vi "processTask.vi"(6 "taskChannelType":T1, 8 "error in (no error)":errorcluster, 11 "classPath":path) -> (0 "error out":errorcluster, 3 "classPath(dup)":path)   [LabVIEW 2023]
uses:
  stopMechanismType.ctl
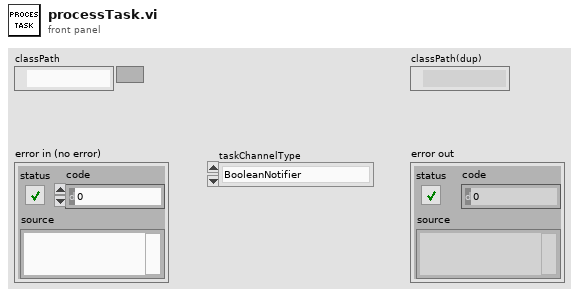
[diagram p1: front panel]
types:
  T1 = typedef "stopMechanismType.ctl" = enum16{"BooleanNotifier", "BooleanUE", "MsgUE", "MsgQueue"}
  T2 = cluster{"placeholderName":string, "filename without extension":string}
  T3 = cluster{"placeholderName":string, "filename without extension":string}[]
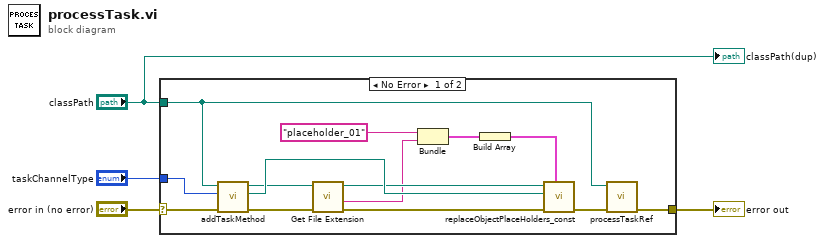
[diagram p0: block diagram]
diagram:
  n1 = case shown="No Error" "error in (no error)" {
    selector: "error in (no error)" -> [w18 w19]
    tunnel: "classPath" -> [w5 _]
    tunnel: [w6 w19] -> w3
    tunnel: "taskChannelType" -> [w15 _]
    frame No Error {
      n2 = call "addTaskMethod.vi"("error in"=w18, "stopMechanismType"=w15, "classPath"=w5) -> ("error out"=w12:errorcluster, "taskViPath"=w16:path, "classPath(dup)"=w10:path)  [unwired: 6 in]
      n3 = call <vilib>:"Get File Extension.vi"("error in (no error)"=w12, "file"=w10) -> ("error out"=w11:errorcluster, "filename without extension"=w8:string, "dup file"=w9:path)  [unwired: 5 in, 2 out]
      n4 = Bundle("placeholderName"="placeholder_01", "filename without extension"=w8) -> (w14:T2)  [unwired: 1 in]
      n5 = Build Array(w14) -> (w13:T3)
      n6 = call "replaceObjectPlaceHolders_const.vi"("placeholderList"=w13, "error in (no error)"=w11, "targetVI"=w16, "classPathToReplace"=w9) -> ("error out"=w7:errorcluster)  [unwired: 7 in]
      n7 = call "processTaskRef.vi"("error in (no error)"=w7, "classPathToReplace"=w5) -> ("error out"=w6:errorcluster)  [unwired: 9 in]
    }
    frame Error {
    }
  }
  "error out" <- w3
  "classPath(dup)" <- "classPath"
